vi "Aero_tunnel_monitor_old.vi"() -> ()   [LabVIEW 2011]
uses:
  Controls/Post_Process.ctl
  <vilib>/Platform/TimedLoop/XDataNode/timing_clust.ctl
  <vilib>/Platform/TimedLoop/XDataNode/nitl_modes.ctl
  <vilib>/Platform/TimedLoop/XDataNode/wakeup.ctl
  ADAM Client/Sub VIs/ADAM Controls/Update_scan_value.ctl
  Globals/Meas_global.vi
  <userlib>/LV-Link3/PolySubVIs/DtCreateAoutChan.vi
  <userlib>/LV-Link3/PolySubVIs/DtOLWriteSingle.vi
  <vilib>/Platform/TimedLoop/XDataNode/XDataNode.xnode
  <vilib>/Platform/TimedLoop/XDataNode/XDNodeRunTimeDep.lvlib
panel:
  in  "Display Graph?":bool
  in  "Menu Ring":u16(ring) items=["Lift", "Pitch", "Drag", "Side", "Yaw", "Roll"]
  in  "Samples":i32=1000
  out "Waveform Chart":dbl[](graph)
  in  "Output Roll":bool
  out "Roll":string="0.0 Nm"
  in  "Output Yaw":bool
  out "Yaw":string="0.0 Nm"
  in  "Output Pitch":bool
  out "Pitch":string="0.0 Nm"
  in  "Output SF":bool
  out "SF":string="0.0 N"
  in  "Output Drag":bool
  out "Drag":string="0.0 N"
  in  "Output Lift":bool
  out "Lift":string="0.0 N"
  in  "Balance Safety limits":T1(array[cluster])=[{"Max +ve Range"=80, "Max -ve Range"=80, "Axis"="Lift"}, {"Max +ve Range"=80, "Max -ve Range"=80, "Axis"="Pitch"}, {"Max +ve Range"=80, "Max -ve Range"=80, "Axis"="Drag"}, {"Max +ve Range"=80, "Max -ve Range"=80, "Axis"="Side-Force"}, {"Max +ve Range"=99, "Max -ve Range"=99, "Axis"="Yaw"}, {"Max +ve Range"=80, "Max -ve Range"=80, "Axis"="Roll"}] {"Max -ve Range" min=0 max=125; "Max +ve Range" min=0 max=125}
  out "Monitor Speed (Hz)":dbl
  out "Belt slip warning":bool
  out "Road Status":string="???"
  in  "GotoYaw":bool
  in  "NewYawPos":dbl
  out "YAW POSITION":dbl
  out "Required WindSpeedRatio":dbl
  out "ROAD SPEED m/s":dbl
  in  "BL Fan1":i32
  in  "BL Fan2":i32
  in  "Stop drive":bool
  in  "Start Drive":bool
  in  "Synch to Wind":bool
  out "Road Info":string="???"
  in  "stop":bool
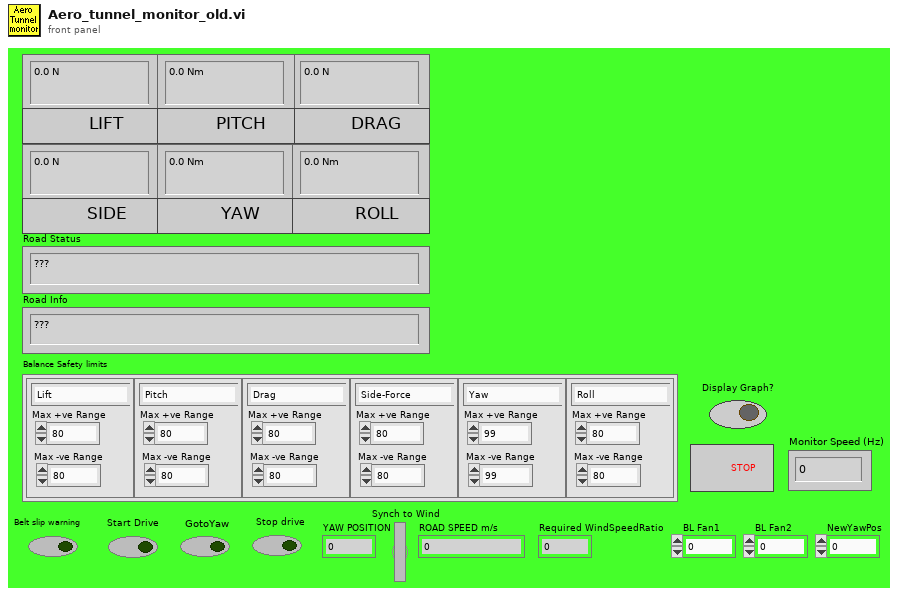
[diagram p1: front panel]
types:
  T1 = cluster{"Max +ve Range":i32, "Max -ve Range":i32, "Axis":string}[]
  T2 = typedef "Post_Process.ctl" = enum16{"Take New Data", "Post Process Raw Data File"}
  T3 = typedef "XDNodeRunTimeDep.lvlib/timing_clust.ctl" = cluster{"Expected End [f-1]":u64, "Actual End [f-1]":u64, "Finished Late? [f-1]":bool, "Expected End [i-1]":u64, "Actual End [i-1]":u64, "Finished Late? [i-1]":bool, "Expected Start [i]":u64, "Actual Start [i]":u64, "Expected Start [f]":u64, "Actual Start [f]":u64, "Source Name":string, "Structure Name":string, "Period":i64, "Deadline":i64, "Offset":i64, "Start":i64, "Priority":i32, "Timeout":i32, "Mode":T4, "Wakeup Reason":T5, "Error":errorcluster, "Source Type":string, "Secondary Source Type":string, "Global End Time":u64, "Global Start Time":u64, "Frame Duration":u64, "Iteration Duration":u64, "Assigned CPU":i32, "I/O Scan Engine Mode":u32}
  T4 = typedef "XDNodeRunTimeDep.lvlib/nitl_modes.ctl" = enum32{"No Change", "Process missed periods, maintain original phase", "Discard missed periods, maintain original phase", "Process missed periods, ignore original phase", "Discard missed periods, ignore original phase"}
  T5 = typedef "XDNodeRunTimeDep.lvlib/wakeup.ctl" = enum32{"Normal", "Aborted", "Asynchronous wakeup", "Timing source error", "Timed loop error", "Timeout"}
  T6 = typedef "Update_scan_value.ctl" = cluster{"Channel Name":string, "New Value":dbl}
  T7 = cluster{"Max +ve Range":i32, "Max -ve Range":i32, "Axis":string}
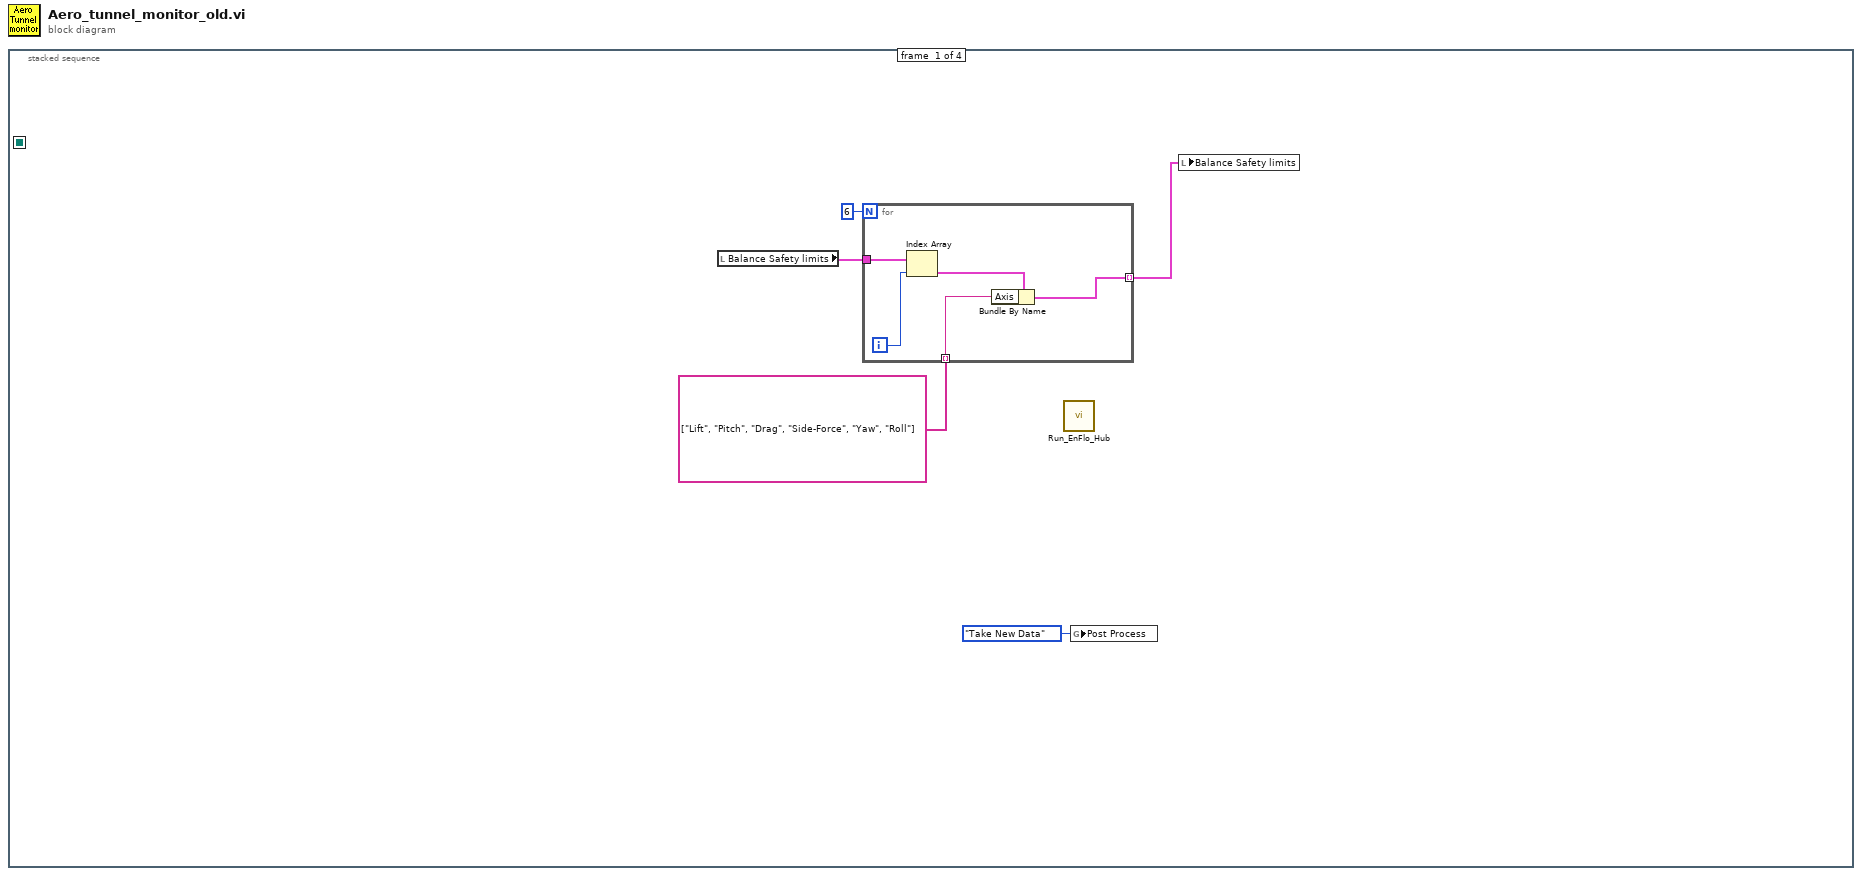
[diagram p0: block diagram]
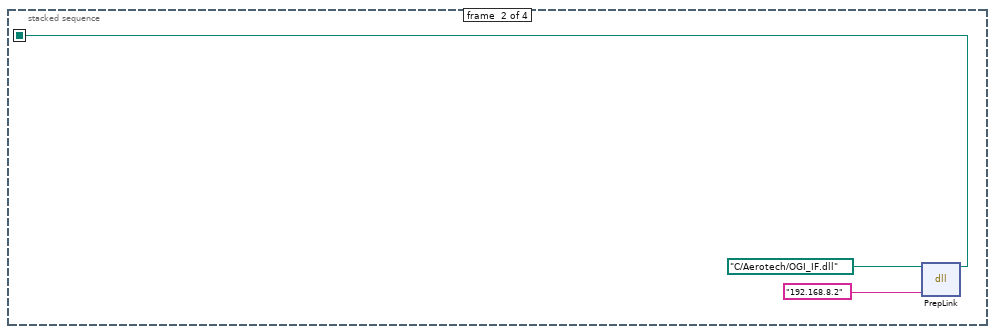
[diagram p2: hidden frame]
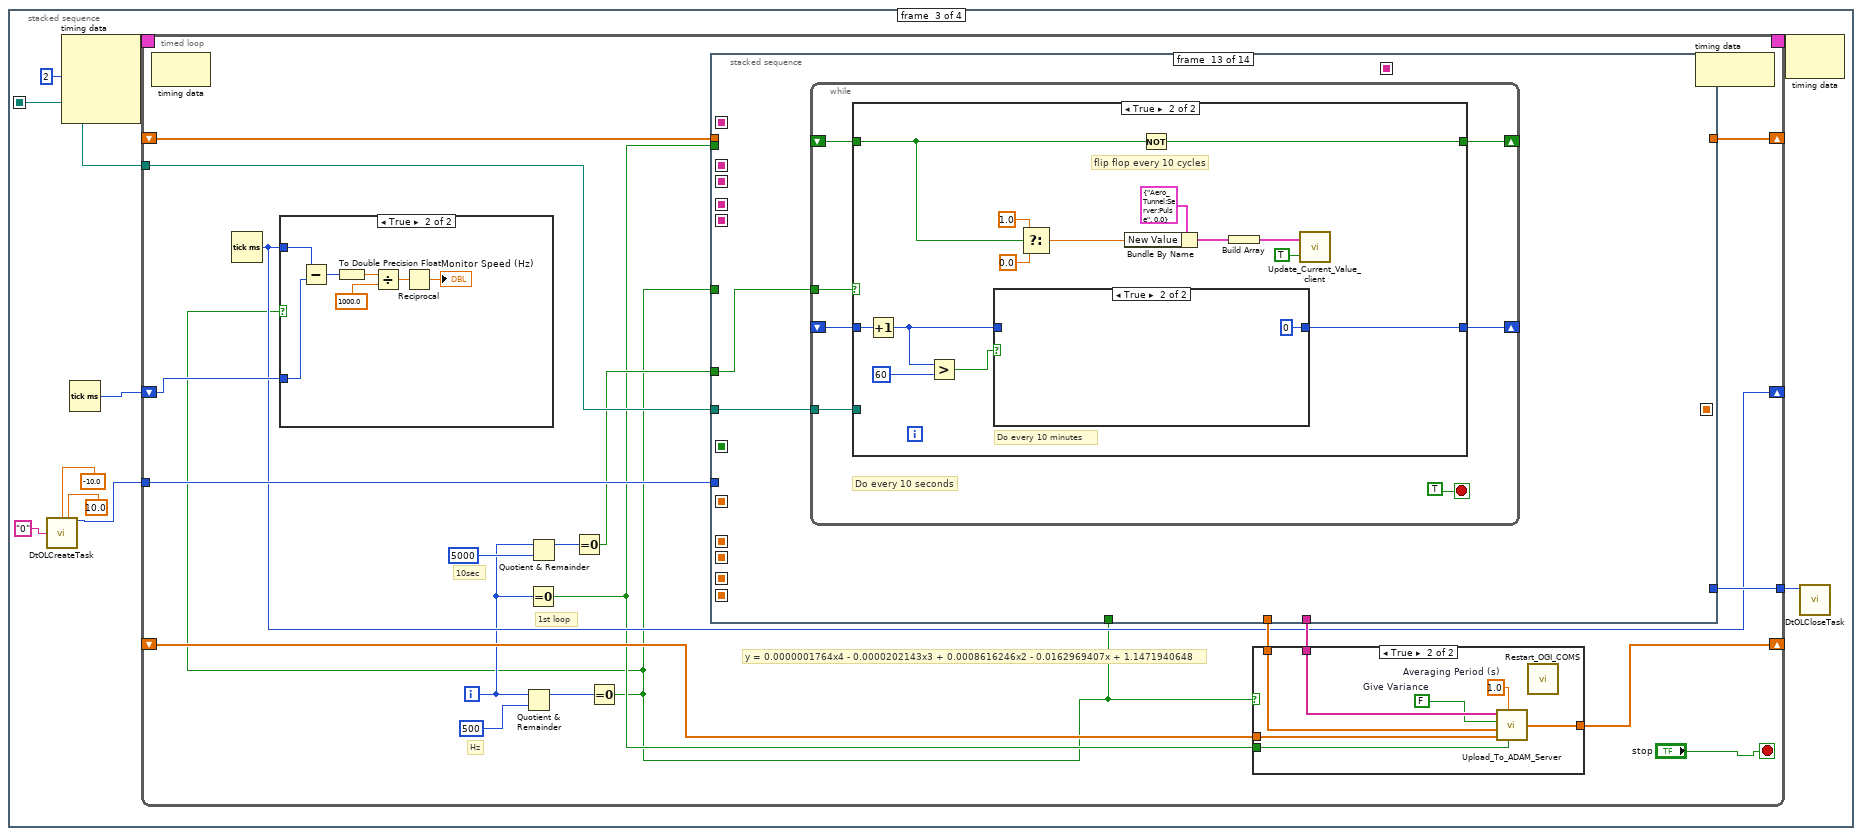
[diagram p3: hidden frame]
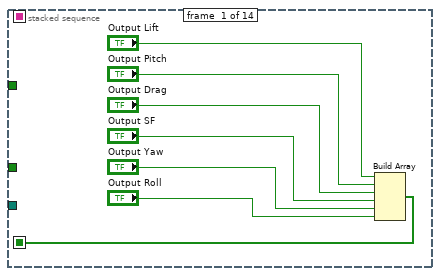
[diagram p6: hidden frame]
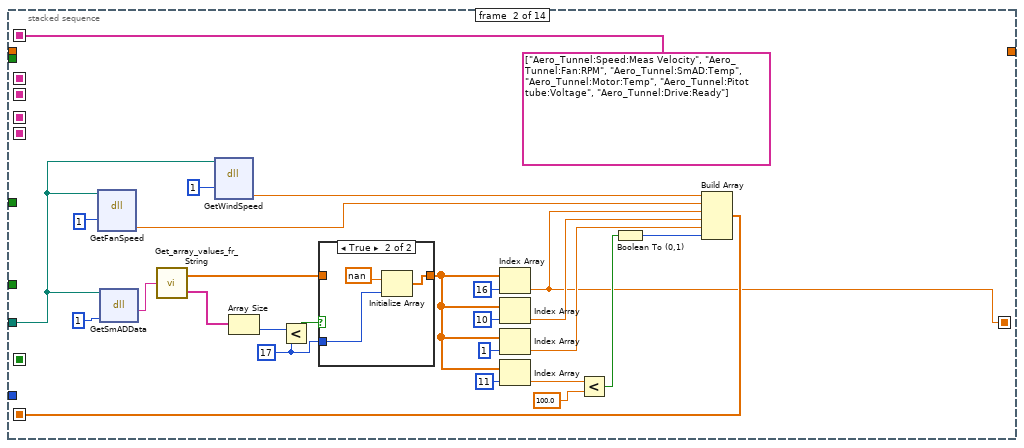
[diagram p7: hidden frame]
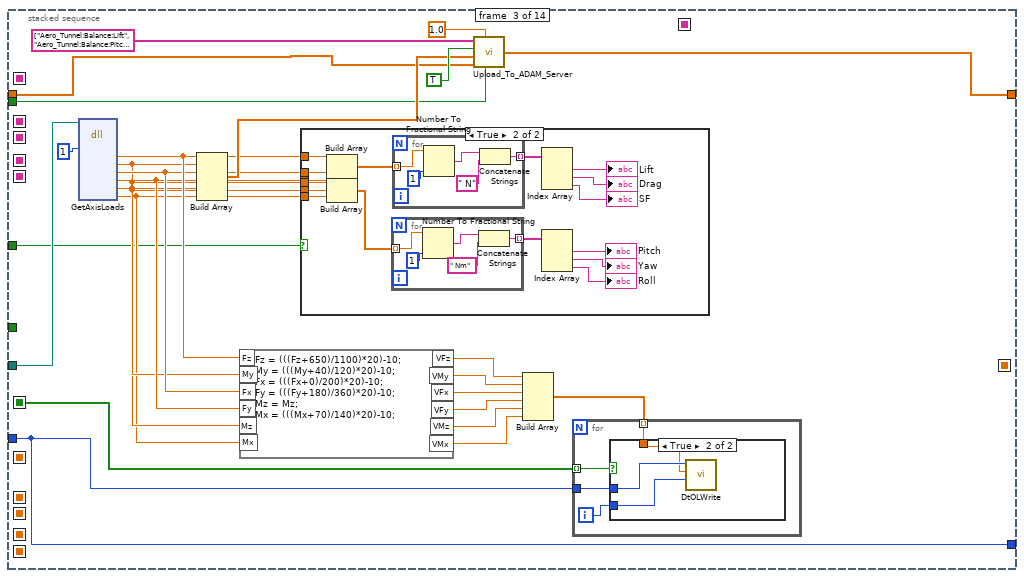
[diagram p9: hidden frame]
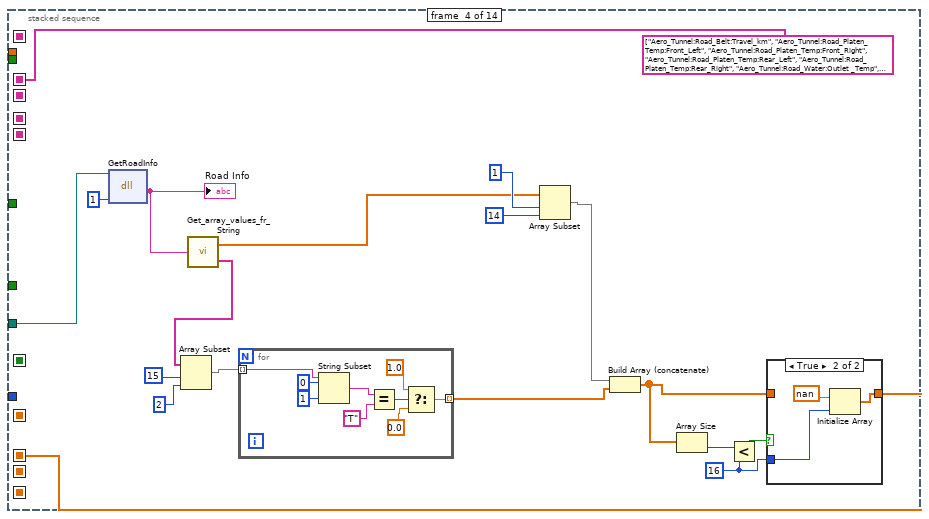
[diagram p12: hidden frame]
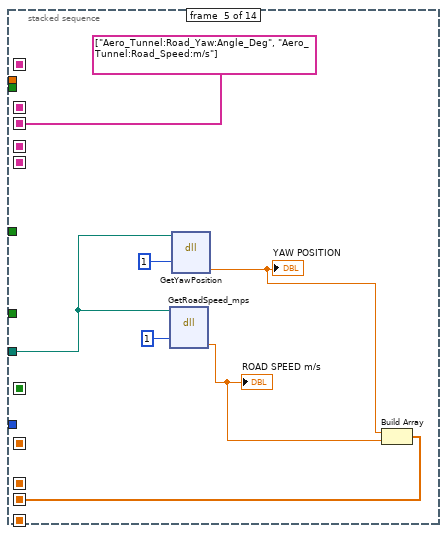
[diagram p14: hidden frame]
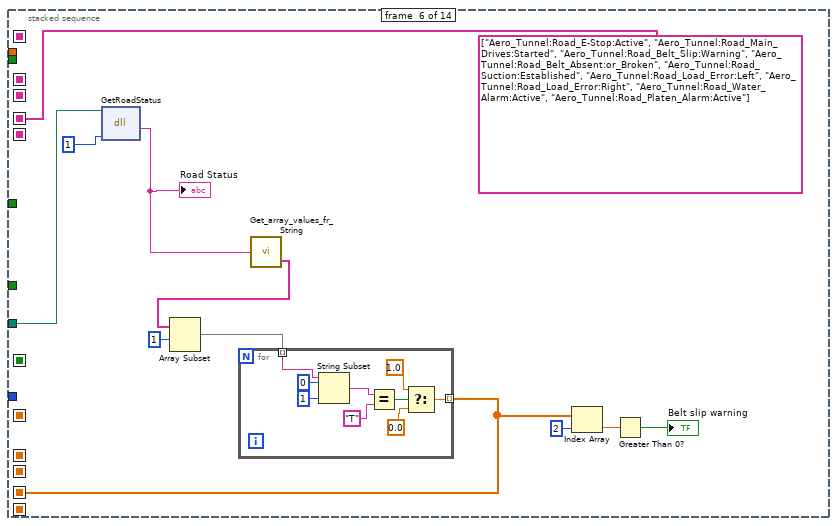
[diagram p15: hidden frame]
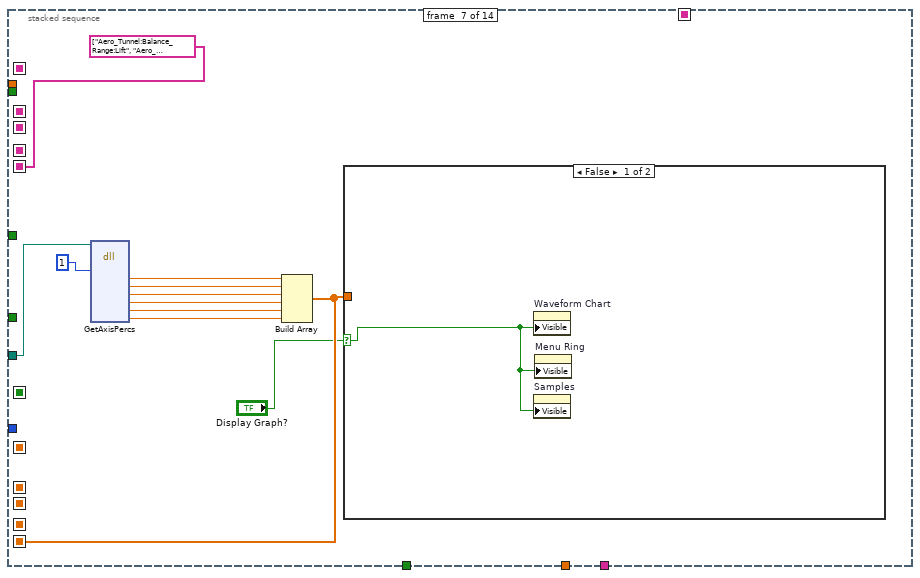
[diagram p16: hidden frame]
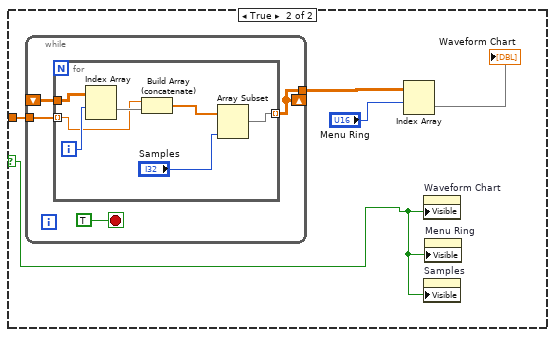
[diagram p17: hidden frame]
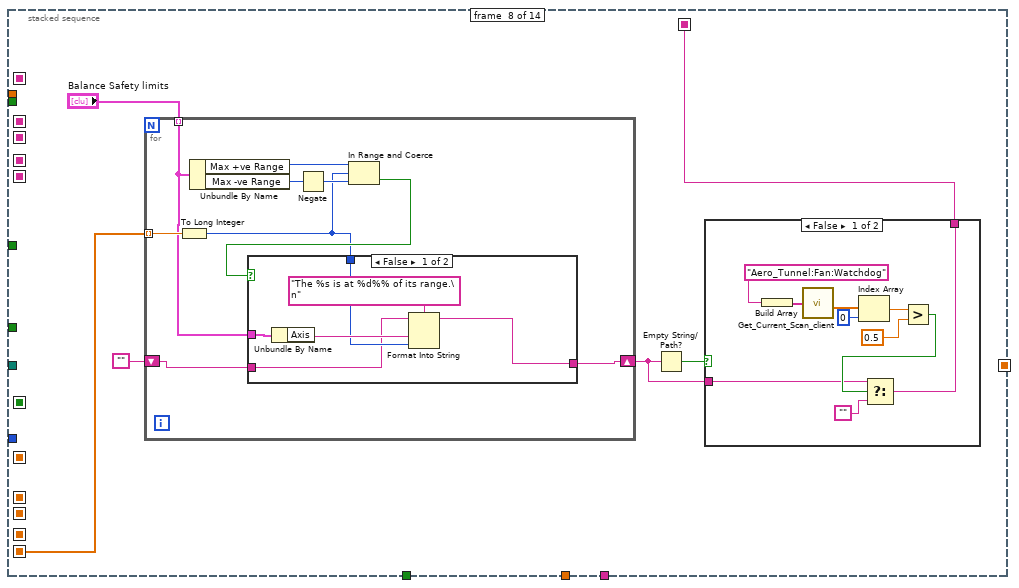
[diagram p18: hidden frame]
diagram:
  n1 = stacked-sequence {
    seq-local: [_ w11 _ _] -> [_ _ w23 w531]
    frame #0 {
      n2 = local read "Balance Safety limits"() -> (w4:T1)
      n3 = for {
        N: 6 -> [_]
        tunnel: w4 -> [w10]
        tunnel: [w7] -> w3 mode=indexing
        tunnel: string[] ["Lift", "Pitch", "Drag", "Side-Force", "Yaw", "Roll"] ("Channel Names") -> [w6] mode=indexing
        i -> [w9]
        n4 = Index Array(array=w10, index=w9) -> (element=w8:T7)
        n5 = Bundle By Name(cluster=w8, "Axis"=w6) -> (w7:T7)
      }
      n6 = call "Run_EnFlo_Hub.vi"() -> ()  [unwired: 8 in]
      n7 = global write "Meas_global.vi" "Post Process"(Post_Process."Take New Data" ("Post Process")) -> ()
      n8 = local write "Balance Safety limits"(w3) -> ()
    }
    frame #1 {
      n9 = dll-call lib="C:/Aerotech/Drivers/OGI_IF.dll" fn="PrepLink"(path in=path "C:/Aerotech/OGI_IF.dll", "IPAddress"="192.168.8.2") -> (path out=w11:path)  [unwired: 2 in, 3 out]
    }
    frame #2 {
      n10 = call-poly <userlib>:"DtOLCreateTask.vi"("Range Min"=-10.0, "Range Max"=10.0, "Channel"="0" ("Channels")) -> ("Task out"=w18:i32)  [unwired: 10 in, 2 out]
      n11 = node-c288(i64 2 ("Period")) -> (w16:T3)  [unwired: 3 in]
      n12 = Tick Count (ms)() -> (millisecond timer value=w22:u32)
      n13 = timed-loop {
        shift-right: [w43] -> _
        shift-left: _ -> [w41]
        tunnel: w23 -> [w39]
        tunnel: [w38] -> w17
        tunnel: w18 -> [w37]
        shift-right: [w35] -> _
        shift-left: _ -> [w36]
        timing: w16 -> [_]
        timing-out: [_] -> w15
        shift-right: [w33] -> _
        shift-left: w22 -> [w34]
        i -> [w27]
        stop <- "stop" stop-if-true
        # "1st loop"
        # "10sec"
        # "Hz"
        # "y = 0.0000001764x4 - 0.0000202143x3 + 0.0008616246x2 - 0.0162969407x + 1.1471940648"
        n14 = node-c288() -> ()  [unwired: 1 in, 1 out]
        n15 = Tick Count (ms)() -> (millisecond timer value=w33:u32)
        n16 = Quotient & Remainder(x=w27, y=500) -> (x-y*floor(x/y)=w30:i32)  [unwired: 1 out]
        n17 = Equal To 0?(x=w27) -> (x = 0?=w26:bool)
        n18 = Quotient & Remainder(x=w27, y=5000) -> (x-y*floor(x/y)=w29:i32)  [unwired: 1 out]
        n19 = Equal To 0?(x=w29) -> (x = 0?=w28:bool)
        n20 = Equal To 0?(x=w30) -> (x = 0?=w25:bool)
        n21 = case shown="True" w25 {
          tunnel: w34 -> [_ w50]
          tunnel: w33 -> [_ w49]
          frame False {
          }
          frame True {
            n22 = Subtract(x=w49, y=w50) -> (x-y=w48:u32)
            n23 = To Double Precision Float(number=w48) -> (double precision float=w44:dbl)
            n24 = Divide(x=w44, y=1000.0) -> (x/y=w46:dbl)
            n25 = Reciprocal(x=w46) -> (1/x=→"Monitor Speed (Hz)":dbl)
          }
        }
        n26 = stacked-sequence {
          seq-local: [_ string[] ["Aero_Tunnel:Speed:Meas Velocity", "Aero_Tunnel:Fan:RPM", "Aero_Tunnel:SmAD:Temp", "Aero_Tunnel:Motor:Temp", "Aero_Tunnel:Pitot tube:Voltage", "Aero_Tunnel:Drive:Ready"] ("Channel Names") _ _ _ _ _ _ _ _ _ _ _ _] -> [_ _ _ _ _ _ _ _ _ _ w331 _ _ _]
          seq-local: [_ w83 _ _ _ _ _ _ _ _ _ _ _ _] -> [_ _ _ _ _ _ _ _ _ _ w330 _ _ _]
          seq-local: [_ _ _ w156 _ _ _ _ _ _ _ _ _ _] -> [_ _ _ _ _ _ _ _ _ _ w327 _ _ _]
          seq-local: [_ _ _ string[] ["Aero_Tunnel:Road_Belt:Travel_km", "Aero_Tunnel:Road_Platen_Temp:Front_Left", "Aero_Tunnel:Road_Platen_Temp:Front_Right", "Aero_Tunnel:Road_Platen_Temp:Rear_Left", "Aero_Tunnel:Road_Platen_Temp:Rear_Right", "Aero_Tunnel:Road_Water:Outlet _Temp", "Aero_Tunnel:Road_Water:Inlet _Temp", "Aero_Tunnel:Road_Suction:Front", "Aero_Tunnel:Road_Suction:Middle", "Aero_Tunnel:Road_Suction:Rear", "Aero_Tunnel:Road_BL_Suction:Primary", "Aero_Tunnel:Road_BL_Suction:Secondary", "Aero_Tunnel:Road_LoadCell:Left", "Aero_Tunnel:Road_LoadCell:Right", "Aero_Tunnel:Road_Water_High:Temp_Alarm", "Aero_Tunnel:Road_Platen_High:Temp_Alarm"] ("Channel Names") _ _ _ _ _ _ _ _ _ _] -> [_ _ _ _ _ _ _ _ _ _ w316 _ _ _]
          seq-local: [_ _ _ _ string[] ["Aero_Tunnel:Road_Yaw:Angle_Deg", "Aero_Tunnel:Road_Speed:m/s"] ("Channel Names") _ _ _ _ _ _ _ _ _] -> [_ _ _ _ _ _ _ _ _ _ w326 _ _ _]
          seq-local: [_ _ _ _ w187 _ _ _ _ _ _ _ _ _] -> [_ _ _ _ _ _ _ _ _ _ w325 _ _ _]
          seq-local: [_ _ _ _ _ string[] ["Aero_Tunnel:Road_E-Stop:Active", "Aero_Tunnel:Road_Main_Drives:Started", "Aero_Tunnel:Road_Belt_Slip:Warning", "Aero_Tunnel:Road_Belt_Absent:or_Broken", "Aero_Tunnel:Road_Suction:Established", "Aero_Tunnel:Road_Load_Error:Left", "Aero_Tunnel:Road_Load_Error:Right", "Aero_Tunnel:Road_Water_Alarm:Active", "Aero_Tunnel:Road_Platen_Alarm:Active"] ("Channel Names") _ _ _ _ _ _ _ _] -> [_ _ _ _ _ _ _ _ _ _ w321 _ _ _]
          seq-local: [_ _ _ _ _ w200 _ _ _ _ _ _ _ _] -> [_ _ _ _ _ _ _ _ _ _ w320 _ _ _]
          seq-local: [w61 _ _ _ _ _ _ _ _ _ _ _ _ _] -> [_ _ w114 _ _ _ _ _ _ _ _ _ _ _]
          seq-local: [_ _ _ _ _ _ string[] ["Aero_Tunnel:Balance_Range:Lift", "Aero_Tunnel:Balance_Range:Pitch", "Aero_Tunnel:Balance_Range:Drag", "Aero_Tunnel:Balance_Range:Side-Force", "Aero_Tunnel:Balance_Range:Yaw", "Aero_Tunnel:Balance_Range:Roll"] ("Channel Names") _ _ _ _ _ _ _] -> [_ _ _ _ _ _ _ _ _ _ w317 _ _ _]
          seq-local: [_ _ _ _ _ _ w215 _ _ _ _ _ _ _] -> [_ _ _ _ _ _ _ w246 _ _ w318 _ _ _]
          seq-local: [_ _ _ _ _ _ _ w242 _ _ _ _ _ _] -> [_ _ _ _ _ _ _ _ w276 w295 _ _ _ _]
          seq-local: [_ w68 _ _ _ _ _ _ _ _ _ _ _ _] -> [_ _ _ _ _ _ _ _ _ w294 _ _ _ _]
          tunnel: [_ _ _ _ _ _ _ _ _ _ w329 _ _ _] -> w42
          tunnel: [_ _ _ _ _ _ _ _ _ _ w328 _ _ _] -> w40
          tunnel: w39 -> [_ w75 w121 w172 w190 w203 w224 _ _ _ w319 w333 w440 w467]
          tunnel: [_ _ w112 _ _ _ _ _ _ _ _ _ _ _] -> w38
          tunnel: w37 -> [_ _ w112 _ _ _ _ _ _ _ _ _ _ _]
          tunnel: w25 -> [_ _ _ _ _ _ _ _ _ _ _ _ _ _]
          tunnel: w36 -> [_ _ w107 _ _ _ _ _ _ _ _ _ _ _]
          tunnel: [_ _ w106 _ _ _ _ _ _ _ _ _ _ _] -> w35
          tunnel: w25 -> [_ _ w99 _ _ _ _ _ _ _ _ w332 _ w466]
          tunnel: w28 -> [_ _ _ _ _ _ _ _ w275 _ _ _ w439 _]
          tunnel: w26 -> [_ _ w98 _ _ _ _ _ _ _ _ _ _ _]
          frame #0 {
            n27 = Build Array("Output Lift", "Output Pitch", "Output Drag", "Output SF", "Output Yaw", "Output Roll") -> (w61:bool[])
          }
          frame #1 {
            w69 = 17 ("y")
            n28 = dll-call lib="C:/Aerotech/Drivers/OGI_IF.dll" fn="GetFanSpeed"(path in=w75, "Enable"=1) -> ("FanSpeedinRPM"=w77:dbl)  [unwired: 3 in, 4 out]
            n29 = dll-call lib="C:/Aerotech/Drivers/OGI_IF.dll" fn="GetSmADData"(path in=w75, "Enable"=1) -> ("SmAD Data String"=w80:string)  [unwired: 2 in, 3 out]
            n30 = call "Get_array_values_fr_String.vi"("String Value"=w80) -> ("Numeric Array"=w70:dbl[], "String array"=w73:string[])
            n31 = dll-call lib="C:/Aerotech/Drivers/OGI_IF.dll" fn="GetWindSpeed"(path in=w75, "Enable"=1) -> ("Windspeed_M/s"=w76:dbl)  [unwired: 3 in, 4 out]
            n32 = Array Size(array=w73) -> (size(s)=w74:i32)
            n33 = Less?(x=w74, y=w69) -> (x < y?=w72:bool)
            n34 = case shown="True" w72 {
              tunnel: [w94 w97] -> w71
              tunnel: w70 -> [w94 _]
              tunnel: w69 -> [_ w95]
              frame False {
              }
              frame True {
                n35 = Initialize Array(nan, w95) -> (w97:dbl[])
              }
            }
            n36 = Index Array(array=w71, index=16) -> (element=w68:dbl)
            n37 = Index Array(array=w71, index=10) -> (element=w91:dbl)
            n38 = Index Array(array=w71, index=1) -> (element=w89:dbl)
            n39 = Index Array(array=w71, index=11) -> (element=w87:dbl)
            n40 = Less?(x=w87, y=100.0) -> (x < y?=w85:bool)
            n41 = Boolean To (0,1)(Boolean=w85) -> (0, 1=w84:i16)
            n42 = Build Array(w76, w77, w68, w91, w89, w84) -> (w83:dbl[])
          }
          frame #2 {
            n43 = dll-call lib="C:/Aerotech/Drivers/OGI_IF.dll" fn="GetAxisLoads"(path in=w121, "Enable"=1) -> ("Lift"=w105:dbl, "Pitch"=w102:dbl, "Drag"=w104:dbl, "side"=w103:dbl, "Yaw"=w101:dbl, "Roll"=w100:dbl)  [unwired: 3 in, 9 out]
            n44 = Build Array(w105, w102, w104, w103, w101, w100) -> (w108:dbl[])
            n45 = formula code="VFz = (((Fz+650)/1100)*20)-10;\nVMy = (((My+40)/120)*20)-10;\nVFx = (((Fx+0)/200)*20)-10;\nVFy = (((Fy+180)/360)*20)-10;\nVMz = Mz;\nVMx = (((Mx+70)/140)*20)-10;"("Fz"=w105, "My"=w102, "Fx"=w104, "Fy"=w103, "Mz"=w101, "Mx"=w100) -> ("VFz"=w120:dbl, "VMy"=w119:dbl, "VFx"=w118:dbl, "VFy"=w117:dbl, "VMz"=w116:dbl, "VMx"=w115:dbl)
            n46 = case shown="True" w99 {
              tunnel: w105 -> [_ w138]
              tunnel: w104 -> [_ w137]
              tunnel: w103 -> [_ w136]
              tunnel: w102 -> [_ w130]
              tunnel: w101 -> [_ w129]
              tunnel: w100 -> [_ w128]
              frame False {
              }
              frame True {
                n47 = Build Array(w138, w137, w136) -> (w135:dbl[])
                n48 = Build Array(w130, w129, w128) -> (w127:dbl[])
                n49 = for {
                  tunnel: w127 -> [w139] mode=indexing
                  tunnel: [w143] -> w126 mode=indexing
                  n50 = Number To Fractional String(number=w139, precision (6)=i16 1) -> (F-format string=w140:string)  [unwired: 2 in]
                  n51 = Concatenate Strings(w140, " Nm" ("string")) -> (w143:string)
                }
                n52 = for {
                  tunnel: w135 -> [w144] mode=indexing
                  tunnel: [w148] -> w134 mode=indexing
                  n53 = Number To Fractional String(number=w144, precision (6)=i16 1) -> (F-format string=w145:string)  [unwired: 2 in]
                  n54 = Concatenate Strings(w145, " N" ("string")) -> (w148:string)
                }
                n55 = Index Array(array=w134) -> (element #1=→"Lift":string, element #2=→"Drag":string, element #3=→"SF":string)  [unwired: 3 in]
                n56 = Index Array(array=w126) -> (element #1=→"Pitch":string, element #2=→"Yaw":string, element #3=→"Roll":string)  [unwired: 3 in]
              }
            }
            n57 = call "Upload_To_ADAM_Server.vi"("First Loop"=w98, "Averaging Period (s)"=1.0, "Shift In"=w107, "Channel Values"=w108, "Give Variance"=TRUE, "Channel Names"=string[] ["Aero_Tunnel:Balance:Lift", "Aero_Tunnel:Balance:Pitch", "Aero_Tunnel:Balance:Drag", "Aero_Tunnel:Balance:Side-Force", "Aero_Tunnel:Balance:Yaw", "Aero_Tunnel:Balance:Roll"]) -> ("Shift Out"=w106:dbl[])
            n58 = Build Array(w120, w119, w118, w117, w116, w115) -> (w113:dbl[])
            n59 = for {
              tunnel: w112 -> [w152]
              tunnel: w114 -> [w151] mode=indexing
              tunnel: w113 -> [w150] mode=indexing
              i -> [w149]
              n60 = case shown="True" w151 {
                tunnel: w152 -> [_ w155]
                tunnel: w150 -> [_ w153]
                tunnel: w149 -> [_ w154]
                frame False {
                }
                frame True {
                  n61 = call-poly <userlib>:"DtOLWrite.vi"("Timeout"=w154, "Data In"=w153, "Task in"=w155) -> ()  [unwired: 7 in, 2 out]
                }
              }
            }
          }
          frame #3 {
            w159 = 16 ("y")
            n62 = dll-call lib="C:/Aerotech/Drivers/OGI_IF.dll" fn="GetRoadInfo"(path in=w172, "Enable"=1) -> ("Road Info"=w171:string)  [unwired: 3 in, 2 out]
            "Road Info" <- w171
            n63 = call "Get_array_values_fr_String.vi"("String Value"=w171) -> ("Numeric Array"=w158:dbl[], "String array"=w162:string[])
            n64 = Array Subset(array=w162, index=15, length=2) -> (w166:string[])
            n65 = for {
              tunnel: w166 -> [w184] mode=indexing
              tunnel: [w178] -> w165 mode=indexing
              n66 = String Subset(string=w184, offset (0)=0, length (rest)=1 ("length (rest)")) -> (substring=w183:string)
              n67 = Equal?(x=w183, y="T") -> (x = y?=w181:bool)
              n68 = Select(t=1.0, s=w181, f=0.0) -> (s? t:f=w178:dbl)
            }
            n69 = Array Subset(array=w158, index=1, length=14) -> (w164:dbl[])
            n70 = Build Array (concatenate)(w164, w165) -> (w157:dbl[])
            n71 = Array Size(array=w157) -> (size(s)=w161:i32)
            n72 = Less?(x=w161, y=w159) -> (x < y?=w160:bool)
            n73 = case shown="True" w160 {
              tunnel: [w174 w177] -> w156
              tunnel: w157 -> [w174 _]
              tunnel: w159 -> [_ w175]
              frame False {
              }
              frame True {
                n74 = Initialize Array(nan, w175) -> (w177:dbl[])
              }
            }
          }
          frame #4 {
            n75 = dll-call lib="C:/Aerotech/Drivers/OGI_IF.dll" fn="GetRoadSpeed_mps"(path in=w190, "Enable"=1) -> ("RoadSpeed_mps"=w188:dbl)  [unwired: 3 in, 4 out]
            "ROAD SPEED m/s" <- w188
            n76 = dll-call lib="C:/Aerotech/Drivers/OGI_IF.dll" fn="GetYawPosition"(path in=w190, "Enable"=1) -> ("Yaw Position"=w189:dbl)  [unwired: 3 in, 4 out]
            "YAW POSITION" <- w189
            n77 = Build Array(w189, w188) -> (w187:dbl[])
          }
          frame #5 {
            n78 = dll-call lib="C:/Aerotech/Drivers/OGI_IF.dll" fn="GetRoadStatus"(path in=w203, "Enable"=1) -> ("Road Status"=w202:string)  [unwired: 3 in, 2 out]
            "Road Status" <- w202
            n79 = call "Get_array_values_fr_String.vi"("String Value"=w202) -> ("String array"=w196:string[])  [unwired: 1 out]
            n80 = Array Subset(array=w196, index=1) -> (w194:string[])  [unwired: 1 in]
            n81 = for {
              tunnel: [w206] -> w200 mode=indexing
              tunnel: w194 -> [w205] mode=indexing
              n82 = String Subset(string=w205, offset (0)=0, length (rest)=1 ("length (rest)")) -> (substring=w211:string)
              n83 = Equal?(x=w211, y="T") -> (x = y?=w209:bool)
              n84 = Select(t=1.0, s=w209, f=0.0) -> (s? t:f=w206:dbl)
            }
            n85 = Index Array(array=w200, index=2) -> (element=w198:dbl)
            n86 = Greater Than 0?(x=w198) -> (x > 0?=→"Belt slip warning":bool)
          }
          frame #6 {
            n87 = dll-call lib="C:/Aerotech/Drivers/OGI_IF.dll" fn="GetAxisPercs"(path in=w224, "Enable"=1) -> ("Lift"=w222:dbl, "Pitch"=w221:dbl, "Drag"=w220:dbl, "side"=w219:dbl, "Yaw"=w218:dbl, "Roll"=w217:dbl)  [unwired: 3 in, 9 out]
            n88 = Build Array(w222, w221, w220, w219, w218, w217) -> (w215:dbl[])
            n89 = case shown="False" "Display Graph?" {
              selector: "Display Graph?" -> [w225 w226]
              tunnel: w215 -> [_ w230]
              frame False {
                n90 = property on="Waveform Chart" class="WFChart (strict)"("Visible"=w225) -> ()  [unwired: 2 in, 2 out]
                n91 = property on="Samples" class="DigNum (strict)"("Visible"=w225) -> ()  [unwired: 2 in, 2 out]
                n92 = property on="Menu Ring" class="Ring (strict)"("Visible"=w225) -> ()  [unwired: 2 in, 2 out]
              }
              frame True {
                n93 = while {
                  shift-right: [w232] -> _
                  shift-left: _ -> [w234]
                  tunnel: w230 -> [w233]
                  tunnel: [w232] -> w229
                  stop <- TRUE stop-if-true
                  n94 = for {
                    tunnel: w234 -> [w237]
                    tunnel: w233 -> [w235] mode=indexing
                    tunnel: [w240] -> w232 mode=indexing
                    i -> [w238]
                    n95 = Index Array(array=w237, index (row)=w238) -> (element=w236:dbl[])  [unwired: 1 in]
                    n96 = Build Array (concatenate)(w235, w236) -> (w241:dbl[])
                    n97 = Array Subset(array=w241, length="Samples") -> (w240:dbl[])  [unwired: 1 in]
                  }
                }
                n98 = Index Array(array=w229, index (row)="Menu Ring") -> (element=→"Waveform Chart":dbl[])  [unwired: 1 in]
                n99 = property on="Waveform Chart" class="WFChart (strict)"("Visible"=w226) -> ()  [unwired: 2 in, 2 out]
                n100 = property on="Samples" class="DigNum (strict)"("Visible"=w226) -> ()  [unwired: 2 in, 2 out]
                n101 = property on="Menu Ring" class="Ring (strict)"("Visible"=w226) -> ()  [unwired: 2 in, 2 out]
              }
            }
          }
          frame #7 {
            n102 = for {
              tunnel: "Balance Safety limits" -> [w262] mode=indexing
              tunnel: w246 -> [w265] mode=indexing
              shift-right: [w259] -> w243
              shift-left: "" -> [w260]
              n103 = To Long Integer(number=w265) -> (32bit integer=w261:i32)
              n104 = Unbundle By Name(w262) -> ("Max +ve Range"=w267:i32, "Max -ve Range"=w266:i32)
              n105 = Negate(x=w266) -> (-x=w264:i32)
              n106 = In Range and Coerce(upper limit=w267, x=w261, lower limit=w264) -> (In Range?=w263:bool)  [unwired: 1 out]
              n107 = case shown="False" w263 {
                tunnel: w262 -> [w273 _]
                tunnel: w261 -> [w271 _]
                tunnel: w260 -> [w269 w274]
                tunnel: [w268 w274] -> w259
                frame False {
                  n108 = Unbundle By Name(w273) -> ("Axis"=w272:string)
                  n109 = Format Into String(format string="The %s is at %d%% of its range.\n", initial string=w269, w272, w271) -> (resulting string=w268:string)  [unwired: 1 in, 1 out]
                }
                frame True {
                }
              }
            }
            n110 = Empty String/Path?(string/path=w243) -> (empty?=w244:bool)
            n111 = case shown="False" w244 {
              tunnel: w243 -> [w250 w258]
              tunnel: [w248 w258] -> w242
              frame False {
                n112 = Build Array("Aero_Tunnel:Fan:Watchdog") -> (w257:string[])
                n113 = call "Get_Current_Scan_client.vi"("ADAM Ch Names"=w257) -> ("Numerical Values"=w255:dbl[])  [unwired: 1 in, 2 out]
                n114 = Index Array(array=w255, index=0) -> (element=w253:dbl)
                n115 = Greater?(x=w253, y=0.5) -> (0:w251:bool)
                n116 = Select(t=w250, s=w251, f="") -> (s? t:f=w248:string)
              }
              frame True {
              }
            }
          }
          frame #8 {
            n117 = while {
              tunnel: w276 -> [w280]
              tunnel: w275 -> [w277]
              stop <- TRUE stop-if-true
              n118 = Empty String/Path?(string/path=w280) -> (empty?=w282:bool)
              n119 = Not(x=w282) -> (.not. x?=w278:bool)
              n120 = Compound Arithmetic op=AND(w278, w277) -> (w281:bool)
              n121 = case shown="True" w281 {
                tunnel: w280 -> [_ w287]
                frame False {
                }
                frame True {
                  w286 = string[] ["Aero_Tunnel:Fan:Watchdog", "Aero_Tunnel:Road:Watchdog", "Aero_Tunnel:Speed:Dem Velocity", "Aero_Tunnel:OGI Dem:Speed"] ("Channel Names")
                  n122 = Format Into String(format string="The Aero Tunnel balance has gone outside of its limits.\n%s\nThe Aero_Tunnel:Fan:Watchdog has therefore been disabled. ", w287) -> (resulting string=w288:string)  [unwired: 2 in, 1 out]
                  n123 = Bundle By Name(cluster=errorcluster {"status"=TRUE, "code"=0, "source"=""} ("error in (no error)"), "source"=w288) -> (w290:errorcluster)
                  n124 = Array Size(array=w286) -> (size(s)=w285:i32)
                  n125 = call "EnFlo_Error_Handler.vi"("error in (no error)"=w290, "Error Type"="Aero Tunnel Balance Range Trip", "Dialog Box (T)"=FALSE) -> ()  [unwired: 3 out]
                  n126 = Initialize Array(0.0, w285) -> (w283:dbl[])
                  n127 = call "ASYNC_Adam_client.vi"("Values"=w283, "Channel Names"=w286) -> ()  [unwired: 2 out]
                }
              }
            }
          }
          frame #9 {
            n128 = while {
              tunnel: w295 -> [_]
              shift-right: [w300] -> _
              shift-left: _ -> [w299]
              tunnel: w294 -> [w297]
              stop <- TRUE stop-if-true
              n129 = Greater?(x=w297, y=35.0) -> (0:w300:bool)
              n130 = Number To Fractional String(number=w297, precision (6)=i16 2) -> (F-format string=w296:string)  [unwired: 2 in]
              n131 = Compound Arithmetic op=AND(invert w299, w300) -> (w303:bool)
              n132 = case shown="True" w303 {
                tunnel: w296 -> [_ w308]
                frame False {
                }
                frame True {
                  w307 = string[] ["Aero_Tunnel:Fan:Watchdog", "Aero_Tunnel:Road:Watchdog", "Aero_Tunnel:Speed:Dem Velocity", "Aero_Tunnel:OGI Dem:Speed"] ("Channel Names")
                  n133 = Format Into String(format string="The Aero Tunnel temperature has gone above it's limits and is:\n%s\nThe Aero_Tunnel:Fan:Watchdog has therefore been disabled. ", w308) -> (resulting string=w309:string)  [unwired: 2 in, 1 out]
                  n134 = Bundle By Name(cluster=errorcluster {"status"=TRUE, "code"=0, "source"=""} ("error in (no error)"), "source"=w309) -> (w311:errorcluster)
                  n135 = Array Size(array=w307) -> (size(s)=w306:i32)
                  n136 = call "EnFlo_Error_Handler.vi"("error in (no error)"=w311, "Error Type"="Aero Tunnel Temperature Trip", "Dialog Box (T)"=FALSE) -> ()  [unwired: 3 out]
                  n137 = Initialize Array(0.0, w306) -> (w304:dbl[])
                  n138 = call "ASYNC_Adam_client.vi"("Values"=w304, "Channel Names"=w307) -> ()  [unwired: 2 out]
                }
              }
            }
          }
          frame #10 {
            n139 = Build Array (concatenate)(w330, w327, w325, w320, w318) -> (w329:dbl[])
            n140 = Boolean To (0,1)(Boolean="GotoYaw") -> (0, 1=w324:i16)
            n141 = Build Array (concatenate)(w331, w316, w326, w321, w317) -> (w328:string[])
            n142 = To Long Integer(number=w324) -> (32bit integer=w315:i32)
            n143 = dll-call lib="C:/Aerotech/Drivers/OGI_IF.dll" fn="GotoYawPosition"(path in=w319, "Enable"=w315, "NewYawPos"="NewYawPos") -> ()  [unwired: 3 in, 4 out]
          }
          frame #11 {
            n144 = case shown="True" w332 {
              selector: w332 -> [_ w334]
              tunnel: w333 -> [_ w335]
              frame False {
              }
              frame True {
                # "Tweak"
                # "Speed"
                # "Tweak"
                # "Speed"
                n145 = stacked-sequence {
                  seq-local: [_ w349 _ _ _ _ _] -> [_ _ _ w389 w403 _ w426]
                  seq-local: [_ w340 _ _ _ _ _] -> [_ _ _ w388 w400 _ _]
                  seq-local: [_ w347 _ _ _ _ _] -> [_ _ _ _ _ w415 _]
                  seq-local: [_ w343 _ _ _ _ _] -> [_ _ _ _ _ _ w428]
                  seq-local: [_ w341 _ _ _ _ _] -> [_ _ _ _ w401 _ _]
                  seq-local: [_ w339 _ _ _ _ _] -> [_ _ _ _ w399 _ _]
                  seq-local: [string[] ["Aero_Tunnel:OGI Dem:Speed", "Froude:NPL:Atmos_Press", "Aero_Tunnel:Motor:Enable", "Aero_Tunnel:Speed:Calib Tweak", "Aero_Tunnel:Upper:Temp", "Aero_Tunnel:Lower:Temp", "Aero_Tunnel:SmAD:Temp", "Aero_Tunnel:Fan:Watchdog"] ("appended array") _ _ _ _ _ _] -> [_ w338 _ _ _ _ _]
                  seq-local: [_ w337 _ _ _ _ _] -> [_ _ w373 _ _ _ _]
                  tunnel: w335 -> [_ w351 _ w387 w402 w414 w429]
                  tunnel: w334 -> [_ _ _ _ _ _ w424]
                  frame #0 {
                  }
                  frame #1 {
                    n146 = call "Get_Current_Scan_client.vi"("ADAM Ch Names"=w338) -> ("Numerical Values"=w337:dbl[])  [unwired: 1 in, 2 out]
                    n147 = Index Array(array=w337, index=0) -> (element=w349:dbl)
                    n148 = Index Array(array=w337, index=3) -> (element=w341:dbl)
                    n149 = Index Array(array=w337, index=1) -> (element=w347:dbl)
                    n150 = while {
                      tunnel: w351 -> [w359]
                      tunnel: w349 -> [w358]
                      shift-right: [w358] -> _
                      shift-left: _ -> [w357]
                      shift-right: [w354] -> _
                      shift-left: _ -> [w355]
                      tunnel: w341 -> [w354]
                      tunnel: [w353] -> w340
                      tunnel: [w352] -> w339
                      stop <- TRUE stop-if-true
                      n151 = Not Equal?(x=w358, y=w357) -> (x != y?=w353:bool)
                      n152 = Not Equal?(x=w354, y=w355) -> (x != y?=w352:bool)
                      n153 = case shown="True" w353 {
                        tunnel: w359 -> [_ w360]
                        tunnel: w358 -> [_ w361]
                        frame False {
                        }
                        frame True {
                          n154 = Greater?(x=w361, y=0.2) -> (0:w362:bool)
                          n155 = Boolean To (0,1)(Boolean=w362) -> (0, 1=w365:i16)
                          n156 = dll-call lib="C:/Aerotech/Drivers/OGI_IF.dll" fn="SetFanSystemState"(path in=w360, "Enable"=1, "Fan ONOFF"=w365) -> ()  [unwired: 3 in, 4 out]
                        }
                      }
                    }
                    n157 = Index Array(array=w337, index=2) -> (element=w345:dbl)
                    n158 = Greater?(x=w345, y=0.5) -> (0:w343:bool)
                  }
                  frame #2 {
                    # "allowed temp."
                    n159 = Index Array(array=w373, index=7) -> (element=w371:dbl)
                    n160 = Array Subset(array=w373, index=4, length=3) -> (w375:dbl[])
                    n161 = Array Max & Min(array=w375) -> (max value=w366:dbl)  [unwired: 3 out]
                    n162 = Greater?(x=w371, y=0.5) -> (0:w368:bool)
                    n163 = Greater?(x=w366, y=35.0) -> (0:w369:bool)
                    n164 = And(x=w369, y=w368) -> (x .and. y?=w367:bool)
                    n165 = case shown="True" w367 {
                      tunnel: w366 -> [_ w380]
                      frame False {
                      }
                      frame True {
                        n166 = Format Into String(format string="Aero Tunnel temp is %.1f. The Aero_Tunnel:Fan:Watchdog has therefore been disabled. ", w380) -> (resulting string=w378:string)  [unwired: 2 in, 1 out]
                        n167 = Bundle By Name(cluster=errorcluster {"status"=TRUE, "code"=0, "source"=""} ("error in (no error)"), "source"=w378) -> (w381:errorcluster)
                        n168 = call "EnFlo_Error_Handler.vi"("error in (no error)"=w381, "Error Type"="Aero Tunnel over temp", "Dialog Box (T)"=FALSE) -> ()  [unwired: 3 out]
                        n169 = call "ASYNC_Adam_client.vi"("Values"=dbl[] [0.0, 0.0], "Channel Names"=string[] ["Aero_Tunnel:Fan:Watchdog", "Aero_Tunnel:Road:Watchdog"]) -> ()  [unwired: 2 out]
                      }
                    }
                  }
                  frame #3 {
                    n170 = case shown="True" w388 {
                      tunnel: w389 -> [_ w396]
                      tunnel: w387 -> [_ w397]
                      frame False {
                      }
                      frame True {
                        n171 = call "Polynomial_convert.vi"("Calib constants"=dbl[] [1.1471940648, -0.0162969407, 0.0008616246, -2.02143e-05, 1.764e-07], "Voltage"=w396) -> ("Eng Values"=w393:dbl)  [unwired: 4 in]
                        n172 = In Range and Coerce(upper limit=1.12, x=w393, lower limit=0.88) -> (coerced(x)=w390:dbl)  [unwired: 1 out]
                        "Required WindSpeedRatio" <- w390
                        n173 = dll-call lib="C:/Aerotech/Drivers/OGI_IF.dll" fn="SetWindSpeedRatio"(path in=w397, "Enable"=1 ("t"), "Required WindSpeedRatio"=w390) -> ()  [unwired: 4 in, 3 out]
                      }
                    }
                  }
                  frame #4 {
                    n174 = Or(x=w400, y=w399) -> (x .or. y?=w398:bool)
                    n175 = case shown="True" w398 {
                      tunnel: w403 -> [_ w408]
                      tunnel: w402 -> [_ w406]
                      tunnel: w401 -> [_ w409]
                      frame False {
                      }
                      frame True {
                        n176 = Divide(x=w409, y=100.0) -> (x/y=w411:dbl)
                        n177 = Increment(x=w411) -> (x+1=w412:dbl)
                        n178 = Multiply(x=w412, y=w408) -> (x*y=w407:dbl)
                        n179 = call "Polynomial_convert.vi"("Calib constants"=dbl[] [36.127, 22.861], "Voltage"=w407) -> ("Eng Values"=w405:dbl)  [unwired: 4 in]
                        n180 = dll-call lib="C:/Aerotech/Drivers/ATE_Surrey_WTCS.dll" fn="SetFanspeed"(path in=w406, "Enable"=1 ("t"), "NewFanSpeed"=w405) -> ()  [unwired: 3 in, 4 out]
                      }
                    }
                  }
                  frame #5 {
                    n181 = while {
                      shift-right: [w417] -> _
                      shift-left: _ -> [w420]
                      tunnel: w415 -> [w417]
                      tunnel: w414 -> [w418]
                      stop <- TRUE stop-if-true
                      n182 = Equal?(x=w417, y=w420) -> (x = y?=w419:bool)
                      n183 = case shown="True" w419 {
                        tunnel: w418 -> [_ w423]
                        tunnel: w417 -> [_ w421]
                        frame False {
                        }
                        frame True {
                          n184 = dll-call lib="C:/Aerotech/Drivers/OGI_IF.dll" fn="SetNewbaroPr_mB"(path in=w423, "Enable"=1, "NewPressure"=w421) -> ()  [unwired: 3 in, 4 out]
                        }
                      }
                    }
                  }
                  frame #6 {
                    n185 = Greater?(x=w426, y=0.1) -> (0:w425:bool)
                    n186 = while {
                      shift-right: [w434] -> _
                      shift-left: _ -> [w433]
                      tunnel: w428 -> [w434]
                      tunnel: w429 -> [w436]
                      tunnel: w425 -> [w432]
                      tunnel: w424 -> [w430]
                      stop <- TRUE stop-if-true
                      n187 = Compound Arithmetic op=AND(w434, invert w433, w432, w430) -> (w431:bool)
                      n188 = case shown="True" w431 {
                        tunnel: w436 -> [_ w438]
                        frame False {
                        }
                        frame True {
                          n189 = dll-call lib="C:/Aerotech/Drivers/OGI_IF.dll" fn="SetPitotZero"(path in=w438, "Enable"=1) -> ()  [unwired: 2 in, 4 out]
                        }
                      }
                    }
                  }
                }
              }
            }
          }
          frame #12 {
            n190 = while {
              tunnel: w440 -> [w447]
              shift-right: [w445] -> _
              shift-left: _ -> [w444]
              tunnel: w439 -> [w443]
              shift-right: [w441] -> _
              shift-left: _ -> [w442]
              stop <- TRUE stop-if-true
              # "Do every 10 seconds"
              n191 = case shown="True" w443 {
                tunnel: w447 -> [_ _]
                tunnel: [w449 w463] -> w445
                tunnel: w444 -> [w449 w462]
                tunnel: w442 -> [w448 w454]
                tunnel: [w448 w452] -> w441
                frame False {
                  (unwired) FALSE
                }
                frame True {
                  # "Do every 10 minutes"
                  # "flip flop every 10 cycles"
                  n192 = Increment(x=w454) -> (x+1=w451:i32)
                  n193 = Greater?(x=w451, y=60) -> (0:w450:bool)
                  n194 = case shown="True" w450 {
                    tunnel: [w464 0] -> w452
                    tunnel: w451 -> [w464 _]
                    frame False {
                    }
                    frame True {
                    }
                  }
                  n195 = Select(t=1.0, s=w462, f=0.0) -> (s? t:f=w456:dbl)
                  n196 = Bundle By Name(cluster=T6 {"Channel Name"="Aero_Tunnel:Server:Pulse", "New Value"=0.0} ("Update Scan Value Cluster"), "New Value"=w456) -> (w458:T6)
                  n197 = Not(x=w462) -> (.not. x?=w463:bool)
                  n198 = Build Array(w458) -> (w457:T6[])
                  n199 = call "Update_Current_Value_client.vi"("Don't Bother with check?"=TRUE, "Update array in"=w457) -> ()
                }
              }
            }
          }
          frame #13 {
            n200 = while {
              shift-right: [w478] -> _
              shift-left: _ -> [w480]
              tunnel: w466 -> [w479]
              tunnel: w467 -> [w476]
              shift-right: [w474] -> _
              shift-left: _ -> [w475]
              shift-right: [w472] -> _
              shift-left: _ -> [w473]
              shift-right: [w469] -> _
              shift-left: _ -> [w471]
              shift-right: [w468] -> _
              shift-left: _ -> [w470]
              stop <- TRUE stop-if-true
              n201 = stacked-sequence {
                tunnel: w480 -> [w486 _ _ _]
                tunnel: w479 -> [w484 w496 w506 w518]
                tunnel: ["Synch to Wind" _ _ _] -> w478
                tunnel: w476 -> [w481 w494 w504 w520]
                tunnel: w475 -> [_ w493 _ _]
                tunnel: [_ "Start Drive" _ _] -> w474
                tunnel: w473 -> [_ _ w503 _]
                tunnel: [_ _ "Stop drive" _] -> w472
                tunnel: w471 -> [_ _ _ w517]
                tunnel: w470 -> [_ _ _ w514]
                tunnel: [_ _ _ "BL Fan1"] -> w469
                tunnel: [_ _ _ "BL Fan2"] -> w468
                frame #0 {
                  n202 = Not Equal?(x="Synch to Wind", y=w486) -> (x != y?=w485:bool)
                  n203 = Or(x=w485, y=w484) -> (x .or. y?=w482:bool)
                  n204 = case shown="True" w482 {
                    tunnel: "Synch to Wind" -> [_ w489]
                    tunnel: w481 -> [_ w488]
                    frame False {
                    }
                    frame True {
                      n205 = Boolean To (0,1)(Boolean=w489) -> (0, 1=w490:i16)
                      n206 = To Long Integer(number=w490) -> (32bit integer=w487:i32)
                      n207 = dll-call lib="C:/Aerotech/Drivers/OGI_IF.dll" fn="RoadSyncToWind"(path in=w488, "Enable"=1, "SynchState"=w487) -> ()  [unwired: 3 in, 4 out]
                    }
                  }
                }
                frame #1 {
                  n208 = Not Equal?(x="Start Drive", y=w493) -> (x != y?=w497:bool)
                  n209 = Or(x=w497, y=w496) -> (x .or. y?=w495:bool)
                  n210 = case shown="True" w495 {
                    tunnel: "Start Drive" -> [_ w501]
                    tunnel: w494 -> [_ w499]
                    frame False {
                    }
                    frame True {
                      n211 = Boolean To (0,1)(Boolean=w501) -> (0, 1=w500:i16)
                      n212 = To Long Integer(number=w500) -> (32bit integer=w498:i32)
                      n213 = dll-call lib="C:/Aerotech/Drivers/OGI_IF.dll" fn="StartRoadDrive"(path in=w499, "Enable"=w498) -> ()  [unwired: 2 in, 4 out]
                    }
                  }
                }
                frame #2 {
                  n214 = Not Equal?(x="Stop drive", y=w503) -> (x != y?=w507:bool)
                  n215 = Or(x=w507, y=w506) -> (x .or. y?=w505:bool)
                  n216 = case shown="True" w505 {
                    tunnel: "Stop drive" -> [_ w511]
                    tunnel: w504 -> [_ w509]
                    frame False {
                    }
                    frame True {
                      n217 = Boolean To (0,1)(Boolean=w511) -> (0, 1=w510:i16)
                      n218 = To Long Integer(number=w510) -> (32bit integer=w508:i32)
                      n219 = dll-call lib="C:/Aerotech/Drivers/OGI_IF.dll" fn="RoadStop"(path in=w509, "Enable"=w508) -> ()  [unwired: 2 in, 4 out]
                    }
                  }
                }
                frame #3 {
                  n220 = Not Equal?(x=w514, y="BL Fan2") -> (x != y?=w515:bool)
                  n221 = Not Equal?(x="BL Fan1", y=w517) -> (x != y?=w516:bool)
                  n222 = Compound Arithmetic op=OR(w516, w515, w518) -> (w519:bool)
                  n223 = case shown="True" w519 {
                    tunnel: w520 -> [_ w522]
                    tunnel: "BL Fan1" -> [_ w524]
                    tunnel: "BL Fan2" -> [_ w523]
                    frame False {
                    }
                    frame True {
                      w521 = 1 ("BL Fan (1 or 2)")
                      n224 = dll-call lib="C:/Aerotech/Drivers/OGI_IF.dll" fn="SetBoundaryPerc"(path in=w522, "enable"=w521, "BL Fan (1 or 2)"=1, "New Percentage"=w524) -> ()  [unwired: 4 in, 4 out]
                      n225 = dll-call lib="C:/Aerotech/Drivers/OGI_IF.dll" fn="SetBoundaryPerc"(path in=w522, "enable"=w521, "BL Fan (1 or 2)"=2, "New Percentage"=w523) -> ()  [unwired: 4 in, 4 out]
                    }
                  }
                }
              }
            }
          }
        }
        n226 = case shown="True" w25 {
          tunnel: [w53 w60] -> w43
          tunnel: w42 -> [_ w59]
          tunnel: w41 -> [w53 w58]
          tunnel: w40 -> [_ w57]
          tunnel: w26 -> [_ w54]
          frame False {
          }
          frame True {
            w55 = FALSE  # Give Variance
            w56 = 1.0  # Averaging Period (s)
            n227 = call "Upload_To_ADAM_Server.vi"("First Loop"=w54, "Averaging Period (s)"=w56, "Shift In"=w58, "Channel Values"=w59, "Give Variance"=w55, "Channel Names"=w57) -> ("Shift Out"=w60:dbl[])
            n228 = call "Restart_OGI_COMS.vi"() -> ()  [unwired: 12 in]
          }
        }
        n229 = node-c288() -> ()  [unwired: 1 in, 1 out]
      }
      n230 = node-c288(w15) -> ()  [unwired: 1 out]
      n231 = call <userlib>:"DtOLCloseTask.vi"("Task in"=w17) -> ()  [unwired: 10 in, 1 out]
    }
    frame #3 {
      n232 = dll-call lib="C:/Aerotech/Drivers/OGI_IF.dll" fn="CloseLink"(path in=w531) -> ()  [unwired: 2 in, 3 out]
    }
  }
